vi "get value.vi"(8 "error in (no error)":errorcluster, 10 "Control Name":string="Pre-Acc", 11 "VI Refnum":refnum<vi>) -> (0 "error out":errorcluster, 2 "get value":ext, 3 "VI Refnum out":refnum<vi>)   [LabVIEW 2016, in "scale sub-VIs.lvlib"]
doc: "Used to get values for 2 set values for a vi"
uses:
  sub-VIs/scale sub-VIs.lvlib
  <vilib>/Utility/Data Type/NI_Data Type.lvlib
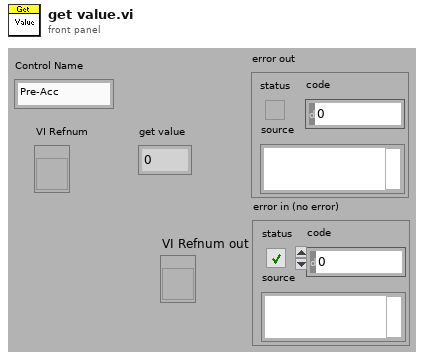
[diagram p1: front panel]
types:
  T1 = typedef "NI_Data Type.lvlib/Data Type.ctl" = enum8{"Invalid Type", "Void", "I8", "I16", "I32", "I64", "U8", "U16", "U32", "U64", "Single Float", "Double Float", "Extended Float", "Single Complex", "Double Complex", "Extended Complex", "Enum U8", "Enum U16", "Enum U32", "Enum U64", "Single Float With Unit", "Double Float With Unit", "Extended Float With Unit", "Single Complex with Unit", "Double Complex with Unit", "Extended Complex with Unit", "Boolean", "String", "Path", "Picture", "Tag", "Array", "Cluster", "Variant", "LV Variant", "Waveform", "Timestamp", "Digital Waveform", "Digital Data", "ExpressData", "Refnum", "External Data", "VI", "Poly VI", "LabVIEW Class Instance", "Fixed Point"}
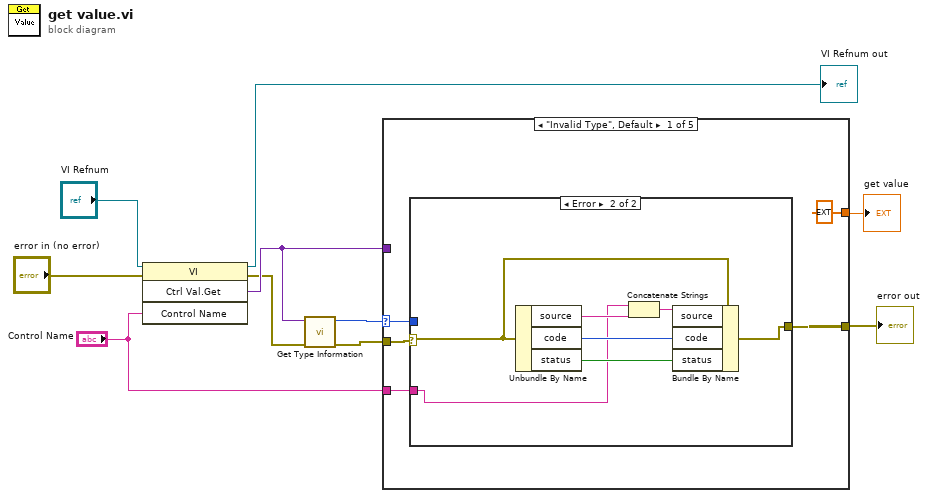
[diagram p0: block diagram]
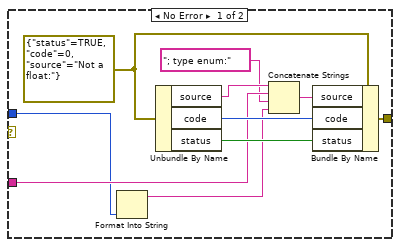
[diagram p2: hidden frame]
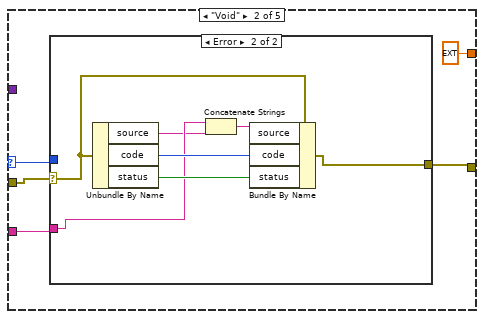
[diagram p3: hidden frame]
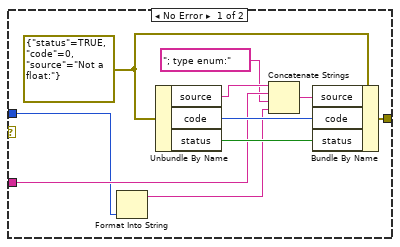
[diagram p4: hidden frame]
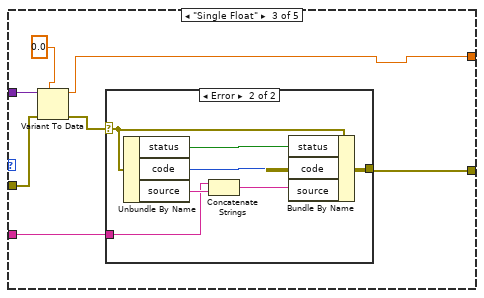
[diagram p5: hidden frame]
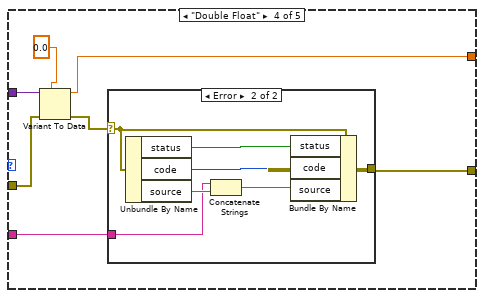
[diagram p7: hidden frame]
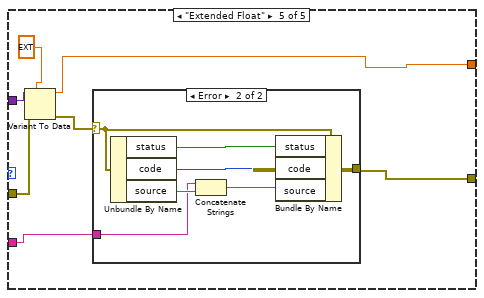
[diagram p9: hidden frame]
diagram:
  n1 = invoke class="VI" method="Ctrl Val.Get"(reference="VI Refnum", error in="error in (no error)", "Control Name"="Control Name") -> (reference out=→"VI Refnum out":refnum<vi>, error out=w3:errorcluster, "Get Control Value Variant"=w4:variant)  [unwired: 1 in, 1 out]
  n2 = call <vilib>:"Get Type Information.vi"("error in (no error)"=w3, "Variant"=w4) -> ("error out"=w2:errorcluster, "Type"=w1:T1)  [unwired: 5 in, 3 out]
  n3 = case shown="\"Invalid Type\", Default" w1 {
    selector: w1 -> [w11 w35 _ _ _]
    tunnel: [ext 0.0 ext 0.0 w59 w76 w89] -> w10
    tunnel: [w15 w36 w58 w74 w88] -> w6
    tunnel: "Control Name" -> [w14 w33 w57 w73 w87]
    tunnel: w4 -> [_ _ w55 w72 w85]
    tunnel: w2 -> [w13 w34 w56 w70 w86]
    frame "Invalid Type", Default {
      n4 = case shown="Error" w13 {
        selector: w13 -> [_ w26]
        tunnel: [w25 w28] -> w15
        tunnel: w14 -> [w20 w27]
        tunnel: w11 -> [w18 _]
        frame No Error {
          w19 = errorcluster {"status"=TRUE, "code"=0, "source"="Not a float:"} ("error constant")
          n5 = Format Into String(w18) -> (resulting string=w17:string)  [unwired: 3 in, 1 out]
          n6 = Unbundle By Name(w19) -> ("source"=w22:string, "code"=w23:i32, "status"=w24:bool)
          n7 = Concatenate Strings(w22, w20, "; type enum:" ("string"), w17) -> (w21:string)
          n8 = Bundle By Name(cluster=w19, "source"=w21, "code"=w23, "status"=w24) -> (w25:errorcluster)
        }
        frame Error {
          n9 = Unbundle By Name(w26) -> ("source"=w29:string, "code"=w31:i32, "status"=w32:bool)
          n10 = Concatenate Strings(w27, w29) -> (w30:string)
          n11 = Bundle By Name(cluster=w26, "source"=w30, "code"=w31, "status"=w32) -> (w28:errorcluster)
        }
      }
    }
    frame "Void" {
      n12 = case shown="Error" w34 {
        selector: w34 -> [_ w51]
        tunnel: [w47 w50] -> w36
        tunnel: w33 -> [w42 w49]
        tunnel: w35 -> [w40 _]
        frame No Error {
          w41 = errorcluster {"status"=TRUE, "code"=0, "source"="Not a float:"} ("error constant")
          n13 = Format Into String(w40) -> (resulting string=w39:string)  [unwired: 3 in, 1 out]
          n14 = Unbundle By Name(w41) -> ("source"=w44:string, "code"=w45:i32, "status"=w46:bool)
          n15 = Concatenate Strings(w44, w42, "; type enum:" ("string"), w39) -> (w43:string)
          n16 = Bundle By Name(cluster=w41, "source"=w43, "code"=w45, "status"=w46) -> (w47:errorcluster)
        }
        frame Error {
          n17 = Unbundle By Name(w51) -> ("source"=w48:string, "code"=w53:i32, "status"=w54:bool)
          n18 = Concatenate Strings(w49, w48) -> (w52:string)
          n19 = Bundle By Name(cluster=w51, "source"=w52, "code"=w53, "status"=w54) -> (w50:errorcluster)
        }
      }
    }
    frame "Single Float" {
      n20 = Variant To Data(error in=w56, type=sgl 0.0, Variant=w55) -> (data=w59:sgl, error out=w61:errorcluster)
      n21 = case shown="Error" w61 {
        selector: w61 -> [w62 w69]
        tunnel: [w62 w66] -> w58
        tunnel: w57 -> [_ w64]
        frame No Error {
        }
        frame Error {
          n22 = Unbundle By Name(w69) -> ("status"=w68:bool, "code"=w67:i32, "source"=w65:string)
          n23 = Concatenate Strings(w64, w65) -> (w63:string)
          n24 = Bundle By Name(cluster=w69, "status"=w68, "code"=w67, "source"=w63) -> (w66:errorcluster)
        }
      }
    }
    frame "Double Float" {
      n25 = Variant To Data(error in=w70, type=0.0, Variant=w72) -> (data=w76:dbl, error out=w75:errorcluster)
      n26 = case shown="Error" w75 {
        selector: w75 -> [w77 w84]
        tunnel: [w77 w81] -> w74
        tunnel: w73 -> [_ w79]
        frame No Error {
        }
        frame Error {
          n27 = Unbundle By Name(w84) -> ("status"=w83:bool, "code"=w82:i32, "source"=w80:string)
          n28 = Concatenate Strings(w79, w80) -> (w78:string)
          n29 = Bundle By Name(cluster=w84, "status"=w83, "code"=w82, "source"=w78) -> (w81:errorcluster)
        }
      }
    }
    frame "Extended Float" {
      n30 = Variant To Data(error in=w86, type=ext 0.0, Variant=w85) -> (data=w89:ext, error out=w91:errorcluster)
      n31 = case shown="Error" w91 {
        selector: w91 -> [w92 w99]
        tunnel: [w92 w96] -> w88
        tunnel: w87 -> [_ w94]
        frame No Error {
        }
        frame Error {
          n32 = Unbundle By Name(w99) -> ("status"=w98:bool, "code"=w97:i32, "source"=w95:string)
          n33 = Concatenate Strings(w94, w95) -> (w93:string)
          n34 = Bundle By Name(cluster=w99, "status"=w98, "code"=w97, "source"=w93) -> (w96:errorcluster)
        }
      }
    }
  }
  "get value" <- w10
  "error out" <- w6
